vi "试验模式表.vi"() -> ()   [LabVIEW 2013]
panel:
  in  "试验模式表":string[](array[string])=["快关L1L2", "快关L1", "快关L2", "步响应1", "归零", "开启关闭", "油压"]
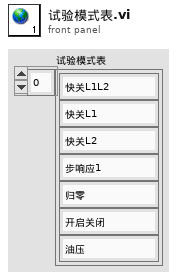
[diagram p1: front panel]
diagram:
